vi "Read Actions.vi"(8 "error in (no error)":errorcluster, 11 "lockin in":refnum<class "system.lvclass">) -> (0 "error out":errorcluster, 2 "Actions":T1, 3 "lockin out":refnum<class "system.lvclass">)   [LabVIEW 2016, in "system.lvclass"]
uses:
  system.lvclass
  Typedefs/lockin_actions.ctl
  system.lvclass/system.ctl
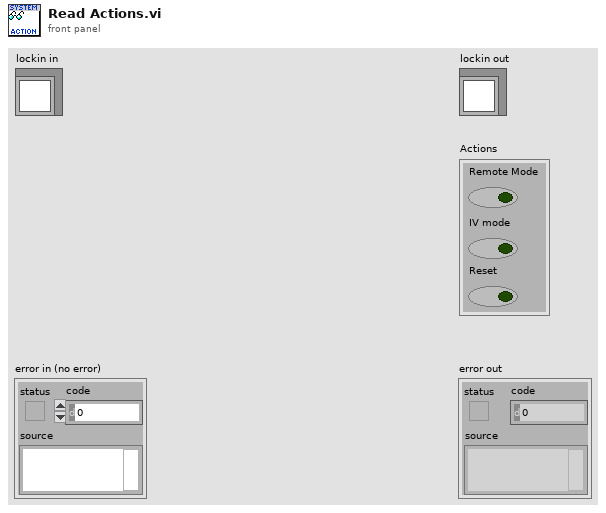
[diagram p1: front panel]
types:
  T1 = typedef "system.lvclass/lockin_actions.ctl" = cluster{"Remote Mode":bool, "IV mode":bool, "Reset":bool}
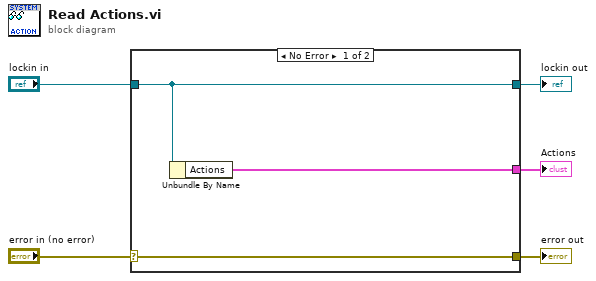
[diagram p0: block diagram]
diagram:
  n1 = case shown="No Error" "error in (no error)" {
    selector: "error in (no error)" -> [w8 w9]
    tunnel: [w8 w9] -> w4
    tunnel: [w7 w10] -> w2
    tunnel: "lockin in" -> [w7 w10]
    tunnel: [w6 _] -> w1
    frame No Error {
      n2 = Unbundle By Name(w7) -> ("Actions"=w6:T1)
    }
    frame Error {
    }
  }
  "error out" <- w4
  "lockin out" <- w2
  "Actions" <- w1
